vi "Indicate Samples.vi"(8 "error in (no error)":errorcluster, 11 "Samples in":refnum<class "Samples.lvclass">) -> (0 "error out":errorcluster, 3 "Samples out":refnum<class "Samples.lvclass">)   [LabVIEW 2015, in "AMS UI.lvlib" / "Samples.lvclass"]
uses:
  Samples.lvclass
  Samples.lvclass/Samples.ctl
  subs/Sample/Sample.lvclass/Sample.ctl
  subs/Sample/Sample.lvclass
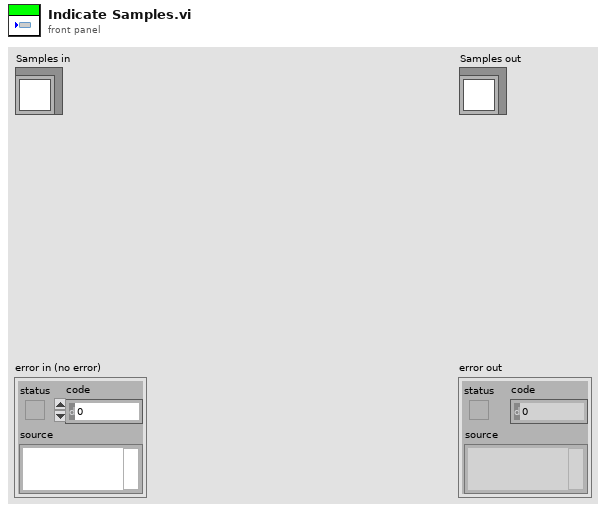
[diagram p1: front panel]
types:
  T1 = typedef "Sample Container.ctl" = cluster{"Sample In":refnum<k21>, "Sample Name":refnum<k21>, "Ti Cathode":refnum<k21>, "SampleQ":refnum<queue>}
  T2 = typedef "FP Control Refs Cluster.ctl" = cluster{"Liquid N Valve References":T3, "Main Line Valve Refs":T4, "Transfer Line Container":refnum<vi>, "Storage Containers":refnum<vi>[], "Sample Refs":T5, "Syringe Ctrl Refs ":T6, "Baratrons Chart":refnum<vi>, "Capillary Container":refnum<vi>, "Preparation Container":refnum<vi>, "Monkey Mode":refnum<vi>}
  T3 = typedef "Liquid N Valve Ref Cluster.ctl" = cluster{"Cold Bath H2O HV 100":refnum<vi>, "Cold Bath Cleaning HV 101":refnum<vi>, "Cold Bath Storage 1 HV 102":refnum<vi>, "Cold Bath Storage 2 HV 103":refnum<vi>, "Cold Bath Storage 3 HV 104":refnum<vi>, "Cold Bath Storage 4 HV 105":refnum<vi>, "Cold Bath Syringe HV 106":refnum<vi>, "Liquid N Master Valve HV 107":refnum<vi>}
  T4 = typedef "Main Line Valve Ref Cluster.ctl" = cluster{"Turbo Valve DV313":refnum<vi>, "Prep Line Valve 0 DV300":refnum<vi>, "Storage Valves":refnum<vi>[]}
  T5 = typedef "Sample Valve Refs.ctl" = cluster{"Valves":cluster{"Sample 5 DV318":refnum<vi>, "Sample 4 DV317":refnum<vi>, "Sample 3 DV316":refnum<vi>, "Sample 2 DV315":refnum<vi>, "Sample 1 DV314":refnum<vi>}, "Lines":cluster{"Sample 1":refnum<vi>, "Sample 2":refnum<vi>, "Sample 3":refnum<vi>, "Sample 4":refnum<vi>, "Sample 5":refnum<vi>}}
  T6 = typedef "Syringe Ctrl Refs.ctl" = cluster{"Syringe Home":refnum<vi>, "Syringe Freeze":refnum<vi>, "Syringe TC":refnum<vi>, "Syringe Container":refnum<vi>}
  T7 = cluster{"Sample 1":refnum<vi>, "Sample 2":refnum<vi>, "Sample 3":refnum<vi>, "Sample 4":refnum<vi>, "Sample 5":refnum<vi>}
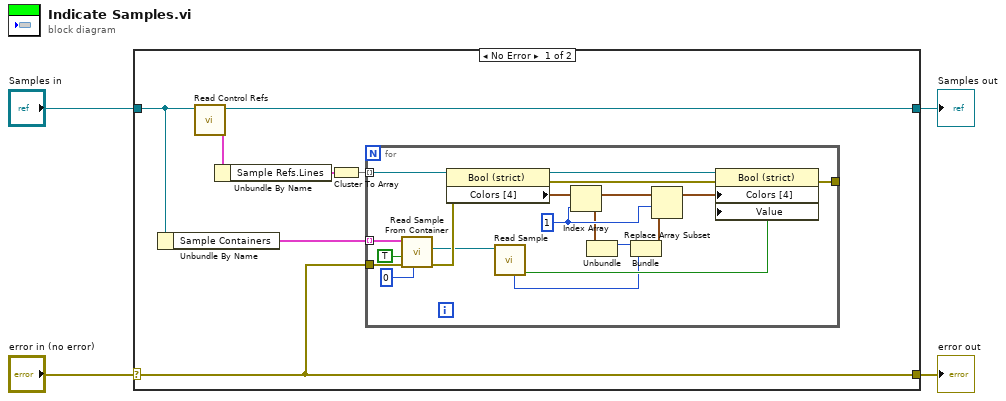
[diagram p0: block diagram]
diagram:
  n1 = case shown="No Error" "error in (no error)" {
    selector: "error in (no error)" -> [w6 w31]
    tunnel: [w6 w31] -> w3
    tunnel: [w9 w30] -> w1
    tunnel: "Samples in" -> [w8 w30]
    frame No Error {
      n2 = Unbundle By Name(w8) -> ("Sample Containers"=w7:T1[])
      n3 = call-dynamic "Read Control Refs.vi"("AMS Gas Actor in"=w8) -> ("Control Refs"=w11:T2, "AMS Gas Actor out"=w9:refnum<class "Samples.lvclass">)  [unwired: 9 in]
      n4 = Unbundle By Name(w11) -> ("Sample Refs.Lines"=w10:T7)
      n5 = Cluster To Array(cluster=w10) -> (array=w5:refnum<vi>[])
      n6 = for {
        tunnel: w5 -> [w29] mode=indexing
        tunnel: [w26] -> _
        tunnel: w7 -> [w19] mode=indexing
        tunnel: w6 -> [w17]
        w24 = 1 ("index")
        n7 = call "Read Sample From Container.vi"("Queue timeout in ms (-1)"=0, "error in (no error)"=w17, "Read from SHV (F)"=TRUE, "Container"=w19) -> ("error out"=w18:errorcluster, "Sample out"=w16:refnum<class "Sample.lvclass">)  [unwired: 3 in, 3 out]
        n8 = property class="Bool (strict)"(reference=w29, error in=w18) -> (reference out=w28:refnum<vi>, error out=w27:errorcluster, "Colors [4]"=w25:cluster{u32, u32}[])
        n9 = call "Read Sample.vi"("Sample in"=w16) -> ("Sample In"=w15:bool, "Color"=w14:u32)  [unwired: 6 in, 3 out]
        n10 = Index Array(array=w25, index=w24) -> (element=w20:cluster{u32, u32})
        n11 = Unbundle(w20) -> (w21:u32)  [unwired: 1 out]
        n12 = Bundle(w21, "Color"=w14) -> (w23:cluster{u32, "Color":u32})  [unwired: 1 in]
        n13 = Replace Array Subset(array=w25, new element=w23, index=w24) -> (w22:cluster{u32, u32}[])
        n14 = property class="Bool (strict)"(reference=w28, error in=w27, "Colors [4]"=w22, "Value"=w15) -> (error out=w26:errorcluster)  [unwired: 1 out]
      }
    }
    frame Error {
    }
  }
  "error out" <- w3
  "Samples out" <- w1
